vi "MsgUsuarioOK.vi"(8 "error in (no error)":errorcluster, 11 "texto":string) -> (0 "error out":errorcluster)   [LabVIEW 2018]
panel:
  in  "OK":bool
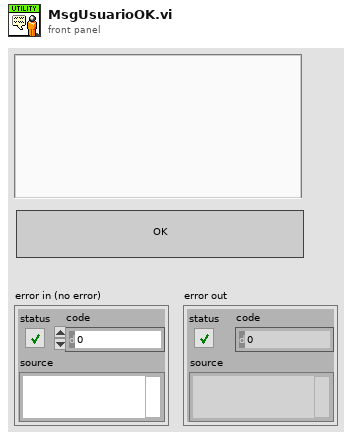
[diagram p1: front panel]
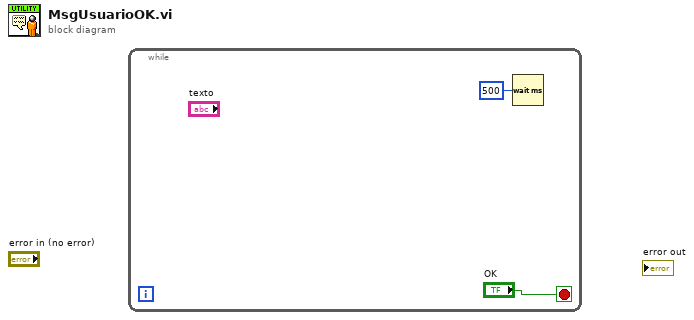
[diagram p0: block diagram]
diagram:
  n1 = while {
    stop <- "OK" stop-if-true
    n2 = Wait (ms)(milliseconds to wait=u32 500) -> ()  [unwired: 1 out]
  }
